vi "VNA_init.vi"(2 "error in (no error)":errorcluster, 3 "VISA name for M9374A":refnum<visa-resource-name>="TCPIP0::WINDOWS-VQFA9LI::hislip0::INSTR") -> (0 "error out":errorcluster, 1 "VISA resource name":refnum<visa-resource-name>)   [LabVIEW 2017]
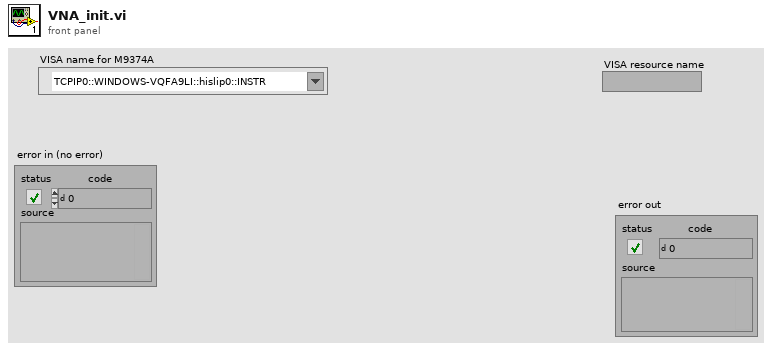
[diagram p1: front panel]
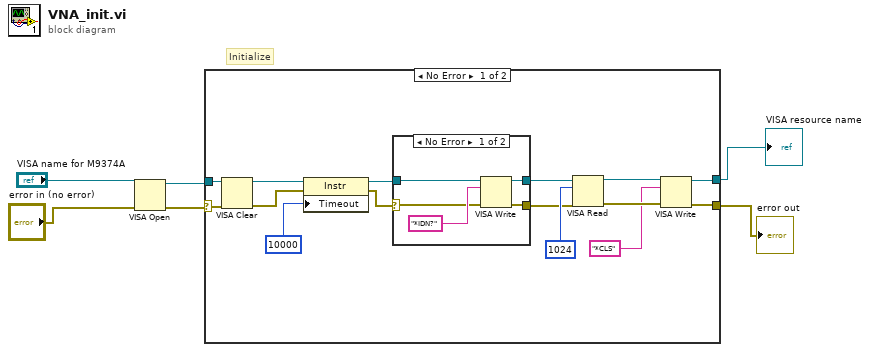
[diagram p0: block diagram]
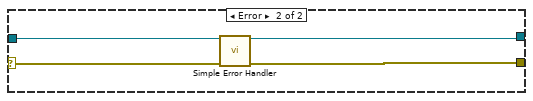
[diagram p3: hidden frame]
diagram:
  # "Initialize"
  n1 = VISA Open(error in (no error)="error in (no error)", VISA resource name="VISA name for M9374A") -> (VISA resource name=w4:refnum<visa-resource-name>, error out=w3:errorcluster)  [unwired: 3 in]
  n2 = case shown="No Error" w3 {
    selector: w3 -> [w21 w31]
    tunnel: [w12 w30] -> w6
    tunnel: [w13 w29] -> w5
    tunnel: w4 -> [w11 w29]
    frame No Error {
      n3 = VISA Clear(VISA resource name=w11, error in (no error)=w21) -> (VISA resource name out=w20:refnum<visa-resource-name>, error out=w19:errorcluster)
      n4 = property class="Instr"(reference=w20, error in=w19, "Timeout"=u32 10000 ("General Settings:Timeout Value")) -> (reference out=w8:refnum<visa-resource-name>, error out=w7:errorcluster)
      n5 = case shown="No Error" w7 {
        selector: w7 -> [w25 w27]
        tunnel: [w23 w27] -> w9
        tunnel: [w24 w28] -> w10
        tunnel: w8 -> [w22 w28]
        frame No Error {
          n6 = VISA Write(VISA resource name=w22, write buffer="*IDN?" ("Cmds"), error in (no error)=w25) -> (VISA resource name out=w24:refnum<visa-resource-name>, error out=w23:errorcluster)  [unwired: 1 out]
        }
        frame Error {
        }
      }
      n7 = VISA Read(VISA resource name=w10, byte count=1024, error in (no error)=w9) -> (VISA resource name out=w16:refnum<visa-resource-name>, error out=w15:errorcluster)  [unwired: 2 out]
      n8 = VISA Write(VISA resource name=w16, write buffer="*CLS" ("Cmds"), error in (no error)=w15) -> (VISA resource name out=w13:refnum<visa-resource-name>, error out=w12:errorcluster)  [unwired: 1 out]
    }
    frame Error {
      n9 = call <vilib>:"Simple Error Handler.vi"("error in (no error)"=w31) -> ("error out"=w30:errorcluster)  [unwired: 4 in, 4 out]
    }
  }
  "VISA resource name" <- w5
  "error out" <- w6
